vi "CreateGraphMenu_OnGraphXaxle.vi"(11 "菜单输入":refnum<k9>) -> ()   [LabVIEW 2015]
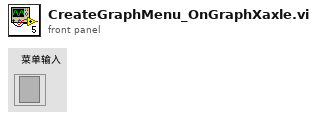
[diagram p1: front panel]
types:
  T1 = cluster{"MenuNames":string[], "MenuTags":string[]}
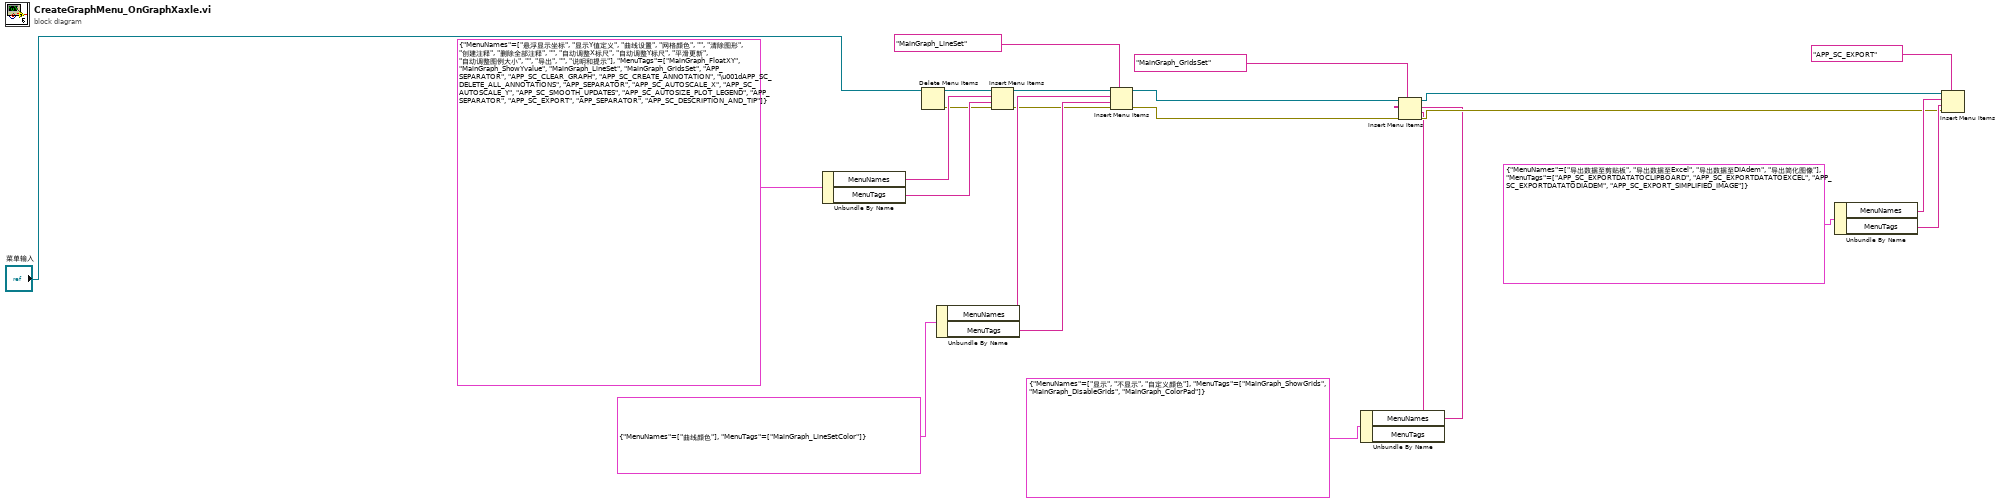
[diagram p0: block diagram]
diagram:
  n1 = Unbundle By Name(T1 {"MenuNames"=["悬浮显示坐标", "显示Y值定义", "曲线设置", "网格颜色", "", "清除图形", "创建注释", "删除全部注释", "", "自动调整X标尺", "自动调整Y标尺", "平滑更新", "自动调整图例大小", "", "导出", "", "说明和提示"], "MenuTags"=["MainGraph_FloatXY", "MainGraph_ShowYvalue", "MainGraph_LineSet", "MainGraph_GridsSet", "APP_SEPARATOR", "APP_SC_CLEAR_GRAPH", "APP_SC_CREATE_ANNOTATION", "\u001dAPP_SC_DELETE_ALL_ANNOTATIONS", "APP_SEPARATOR", "APP_SC_AUTOSCALE_X", "APP_SC_AUTOSCALE_Y", "APP_SC_SMOOTH_UPDATES", "APP_SC_AUTOSIZE_PLOT_LEGEND", "APP_SEPARATOR", "APP_SC_EXPORT", "APP_SEPARATOR", "APP_SC_DESCRIPTION_AND_TIP"]}) -> ("MenuNames"=w10:string[], "MenuTags"=w11:string[])
  n2 = Delete Menu Items(9:"菜单输入") -> (0:w1:errorcluster, 3:w4:refnum<k9>)  [unwired: 3 in]
  n3 = Unbundle By Name(T1 {"MenuNames"=["曲线颜色"], "MenuTags"=["MainGraph_LineSetColor"]}) -> ("MenuNames"=w14:string[], "MenuTags"=w13:string[])
  n4 = Insert Menu Items(6:w1, 7:w11, 8:w10, 9:w4) -> (0:w3:errorcluster, 3:w8:refnum<k9>)  [unwired: 2 in, 1 out]
  n5 = Insert Menu Items(5:"MainGraph_LineSet" ("L10n_menu tag"), 6:w3, 7:w13, 8:w14, 9:w8) -> (0:w2:errorcluster, 3:w7:refnum<k9>)  [unwired: 1 in, 1 out]
  n6 = Unbundle By Name(T1 {"MenuNames"=["显示", "不显示", "自定义颜色"], "MenuTags"=["MainGraph_ShowGrids", "MainGraph_DisableGrids", "MainGraph_ColorPad"]}) -> ("MenuNames"=w16:string[], "MenuTags"=w17:string[])
  n7 = Insert Menu Items(5:"MainGraph_GridsSet" ("L10n_menu tag"), 6:w2, 7:w17, 8:w16, 9:w7) -> (0:w19:errorcluster, 3:w20:refnum<k9>)  [unwired: 1 in, 1 out]
  n8 = Unbundle By Name(T1 {"MenuNames"=["导出数据至剪贴板", "导出数据至Excel", "导出数据至DIAdem", "导出简化图像"], "MenuTags"=["APP_SC_EXPORTDATATOCLIPBOARD", "APP_SC_EXPORTDATATOEXCEL", "APP_SC_EXPORTDATATODIADEM", "APP_SC_EXPORT_SIMPLIFIED_IMAGE"]}) -> ("MenuNames"=w23:string[], "MenuTags"=w24:string[])
  n9 = Insert Menu Items(5:"APP_SC_EXPORT" ("L10n_menu tag"), 6:w19, 7:w24, 8:w23, 9:w20) -> ()  [unwired: 1 in, 3 out]
